vi "Write Data to TDMS File Core.vi"(8 "error in (no error)":errorcluster, 10 "TDMS-Container":refnum<class "TDMS-Container.lvclass">, 11 "TDMS-Actor in":refnum<class "TDMS-Actor.lvclass">=refnum) -> (0 "error out":errorcluster, 3 "TDMS-Actor out":refnum<class "TDMS-Actor.lvclass">)   [LabVIEW 2016, in "BNT_TDMS.lvlib" / "TDMS-Actor.lvclass"]
doc: "Write TDMS-Container to file.\n\n<b>Attention:</b> This is a dynamich dispatch VI to be overitten by derived classes. A default implementation maybe add later."
uses:
  TDMS-Actor.lvclass
  TDMSContainer/TDMS-Container.lvclass
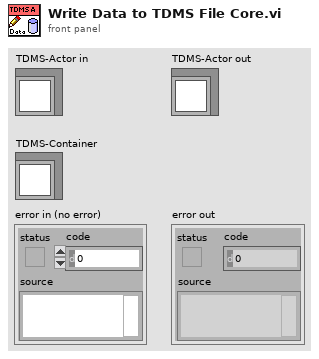
[diagram p1: front panel]
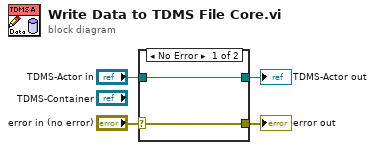
[diagram p0: block diagram]
diagram:
  n1 = case shown="No Error" "error in (no error)" {
    selector: "error in (no error)" -> [w5 w8]
    tunnel: [w5 w8] -> w3
    tunnel: [w6 w7] -> w1
    tunnel: "TDMS-Actor in" -> [w6 w7]
    frame No Error {
    }
    frame Error {
    }
  }
  "error out" <- w3
  "TDMS-Actor out" <- w1
